vi "InflationApparatus.vi"() -> ()   [LabVIEW 2020]
uses:
  Controls/Outputs.ctl
  <vilib>/userDefined/High Color/IMAQdx.ctl
  Controls/Serpoint.ctl
  Controls/BR2.ctl
  Controls/ButtonEnum.ctl
  Controls/TFspec.ctl
  Controls/Calibration.ctl
  <vilib>/Analysis/6fits.llb/Curve Fitting Criteria.ctl
  <vilib>/DAQmx/read.llb/DAQmx Read (Analog 1D DBL 1Chan NSamp).vi
  <extravilib>/ChannelInstances/Tag-bool/Read With Abort.vi
  <extravilib>/ChannelInstances/Tag-bool/Write With Abort.vi
  <extravilib>/ChannelInstances/Tag-bool/Instantiate.vi
  <extravilib>/ChannelInstances/Tag-bool/EndpointRead.vi
  <extravilib>/ChannelInstances/Tag-bool/Endpoint.vi
  <vilib>/DAQmx/create/channels.llb/DAQmx Create Channel (AI-Voltage-Basic).vi
  <vilib>/DAQmx/configure/timing.llb/DAQmx Timing (Sample Clock).vi
  <vilib>/DAQmx/miscellaneous.llb/DAQmx Fill In Error Info.vi
  <vilib>/Analysis/NI_AALPro.lvlib
  <extravilib>/ChannelInstances/Tag-bool.lvlib
panel:
  in  "Program Stop":bool
  in  "Tab Control":T1(tab)
  in  "Inputs":T4={"File Name"="test.txt", "Force (Hz)"=30.0, "Camera (Hz)"=30.0, "Systole (V)"=0.5, "Diastole (V)"=0.2, "T (sec)"=10.0, "Delay (sec)"=2.0, "Setpoint Function"=enum."Ramp", "Max Diam (mm)"=70.0, "DAQmx Servo Task"="MyPulseOutputTask", "Force Sensor Channel"="Dev2/ai7", "DAQmx LED Task"="MyDigitalOutTask", "Camera Selector"="cam5", "FS Task Out"="", "Servo Task Out"="", "LED Task Out"="", "Camera Session Out"="", "Color Pane"=0} {"Color Pane" items=["Blue", "Red", "Green", "Saturation", "Value", "Intensity", "Luminance", "Hue", ""]}
  in  "ANALYZE":bool
  in  "WRITE TO FILE":bool
  out "Start Time":timestamp
  out "Camera Framerate":dbl(knob) scale=0.0..50.0
  in  "CLEAR \nCHARTS":bool
  in  "Main Start":bool
  out "Diameter (mm)":dbl(graph)
  out "Force Output vs. Setpoint (in Volts)":cluster{"Force Setpoint":dbl, "Force Value":dbl}(graph)
  in  "Main Stop":bool
  out "Camera Buffer":u32
  out "R-Squared":dbl
  out "Outputs":T5
  out "unPWM Signal":dbl[](array[numeric])
  in  "FC Stop":bool
  in  "FC Calculate":bool
  in  "FC Start":bool
  out "Force Sensor Output":dbl(graph)
  in  "FC Log":bool
  out "Calibration Equations":string[][](table)
  out "Calibration Values":string[][](table)
  in  "DAQ Channel":tag="Dev2/ai7"
  in  "Camera Collect":bool
  out "Image":T6(plugin-control)
  in  "Camera Selector":T3
  in  "Settings \n(Clamp (Rake))":T7={"Contrast"=16, "Filter width"=10, "Steepness"=63, "Subsampling Ratio"=30, "Show Search Area"=TRUE, "Show Search Lines"=TRUE, "Show Edges Found"=TRUE, "Show Result"=TRUE}
  out "Framerate":dbl(knob)=4.995836802664447 scale=0.0..100.0
  out "Buffer Number Out":u32=363
  out "Diam (mm)":dbl
  in  "Color Plane":i32(ring)=2 items=["Red", "Green", "Blue", "Hue", "Saturation", "Luminance", "Value", "Intensity"]
  # "Test Variables:"
  # "Sampling Frequencies:"
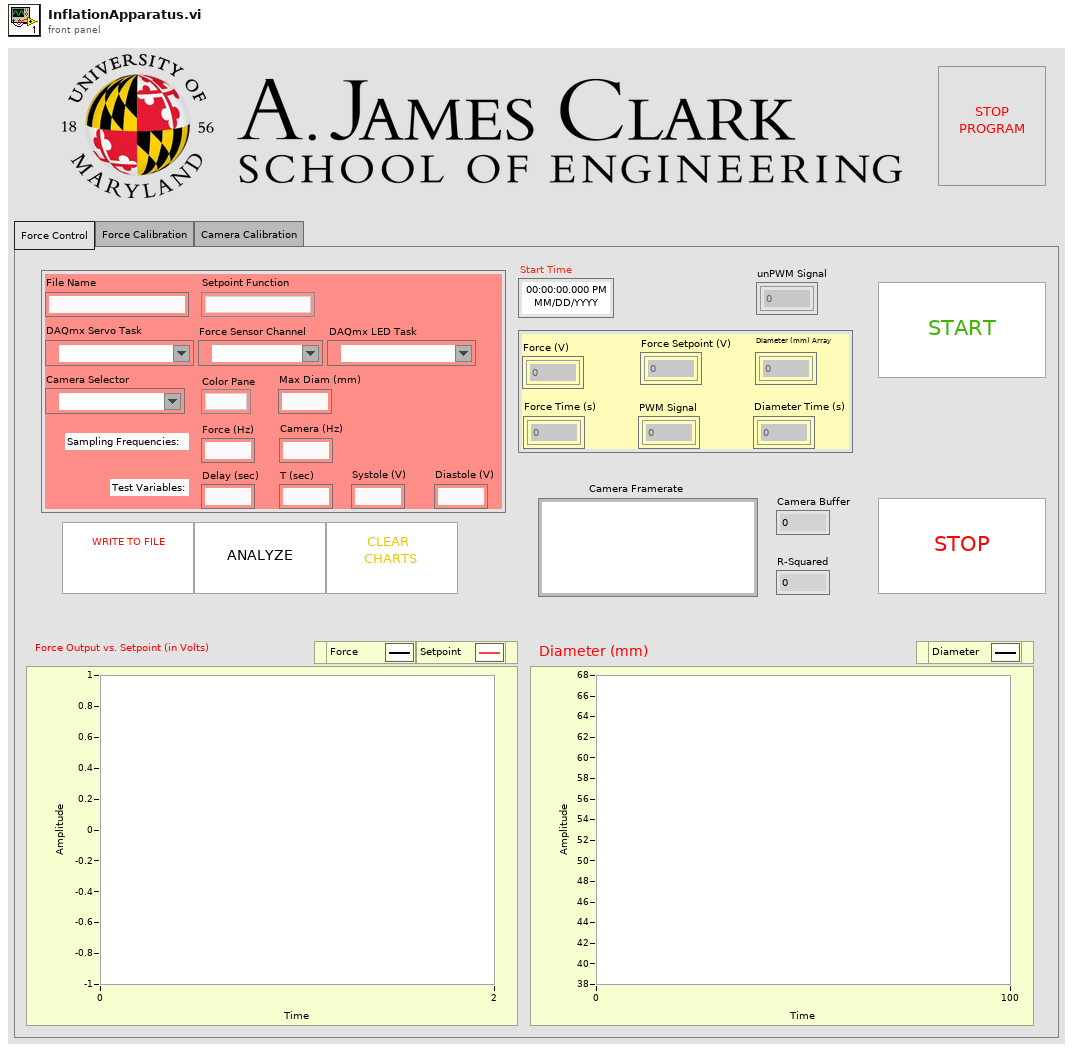
[diagram p1: front panel]
types:
  T1 = enum32{"Force Control", "Force Calibration", "Camera Calibration"}
  T2 = typedef "Serpoint.ctl" = enum16{"Incremental PWM Step", "PWM Step", "Ramp", "Sinusoidal", "Blood-Pressure"}
  T3 = typedef "IMAQdx.ctl" = refnum<k21>
  T4 = cluster{"File Name":string, "Force (Hz)":dbl, "Camera (Hz)":dbl, "Systole (V)":dbl, "Diastole (V)":dbl, "T (sec)":dbl, "Delay (sec)":dbl, "Setpoint Function":T2, "Max Diam (mm)":dbl, "DAQmx Servo Task":refnum<k21>, "Force Sensor Channel":tag, "DAQmx LED Task":refnum<k21>, "Camera Selector":T3, "FS Task Out":refnum<k21>, "Servo Task Out":refnum<k21>, "LED Task Out":refnum<k21>, "Camera Session Out":T3, "Color Pane":i32}
  T5 = typedef "Outputs.ctl" = cluster{"Force Setpoint (V)":dbl[], "PWM Signal":dbl[], "Diameter (mm) Array":dbl[], "Force (V)":dbl[], "Diameter Time (s)":dbl[], "Force Time (s)":dbl[]}
  T6 = typedef "IMAQ Image.ctl" = refnum<image>
  T7 = cluster{"Contrast":i32, "Filter width":i32, "Steepness":i32, "Subsampling Ratio":u32, "Show Search Area":bool, "Show Search Lines":bool, "Show Edges Found":bool, "Show Result":bool}
  T8 = typedef "ButtonEnum.ctl" = enum16{"Initialize", "Analyze", "Clear Charts", "Write to File", "Main Start", "Force Calibration Start", "Force Calibration Calibrate", "Camera Calibration", "Program Stop"}
  T9 = typedef "BR2.ctl" = cluster{"Analyze":refnum<vi>, "Write to File":refnum<vi>, "Clear Charts":refnum<vi>}
  T10 = enum8{"Enabled", "Disabled", "Disabled and Grayed Out"}
  T11 = typedef "TFspec.ctl" = cluster{"b0":dbl, "b1":dbl, "b2":dbl, "a0":dbl, "a1":dbl, "a2":dbl}
  T12 = cluster{"Force Setpoint":dbl, "Force Value":dbl}[]
  T13 = typedef "Inputs.ctl" = cluster{"File Name":string, "Force (Hz)":dbl, "Camera (Hz)":dbl, "Systole (V)":dbl, "Diastole (V)":dbl, "T (sec)":dbl, "Delay (sec)":dbl, "Setpoint Function":T2, "Max Diam (mm)":dbl, "DAQmx Servo Task":refnum<k21>, "Force Sensor Channel":tag, "DAQmx LED Task":refnum<k21>, "Camera Selector":T3, "FS Task Out":refnum<k21>, "Servo Task Out":refnum<k21>, "LED Task Out":refnum<k21>, "Camera Session Out":T3, "Color Pane":i32}
  T14 = typedef "controlspec.ctl" = cluster{"Transfer Function":cluster{"Numerator":dbl[], "Denominator":dbl[]}, "Limit Cluster":cluster{"Upper Limit":dbl, "Lower Limit":dbl}}
  T15 = typedef "ForceCluster.ctl" = cluster{"Force Setpoint":dbl, "PWM Signal":dbl, "Force Value":dbl, "UnPWM Signal":dbl}
  T16 = typedef "Tag-bool.lvlib/))Channel.ctl" = refnum<queue>
  T17 = cluster{"Camera Framerate":dbl, "Camera Buffer":u32, "Diameter (mm)":dbl}
  T18 = typedef "Calibration.ctl" = cluster{"R^2":dbl[], "b":dbl[], "m":dbl[], "CalTable":string[][]}
  T19 = typedef "NI_AALPro.lvlib/Curve Fitting Criteria.ctl" = u16
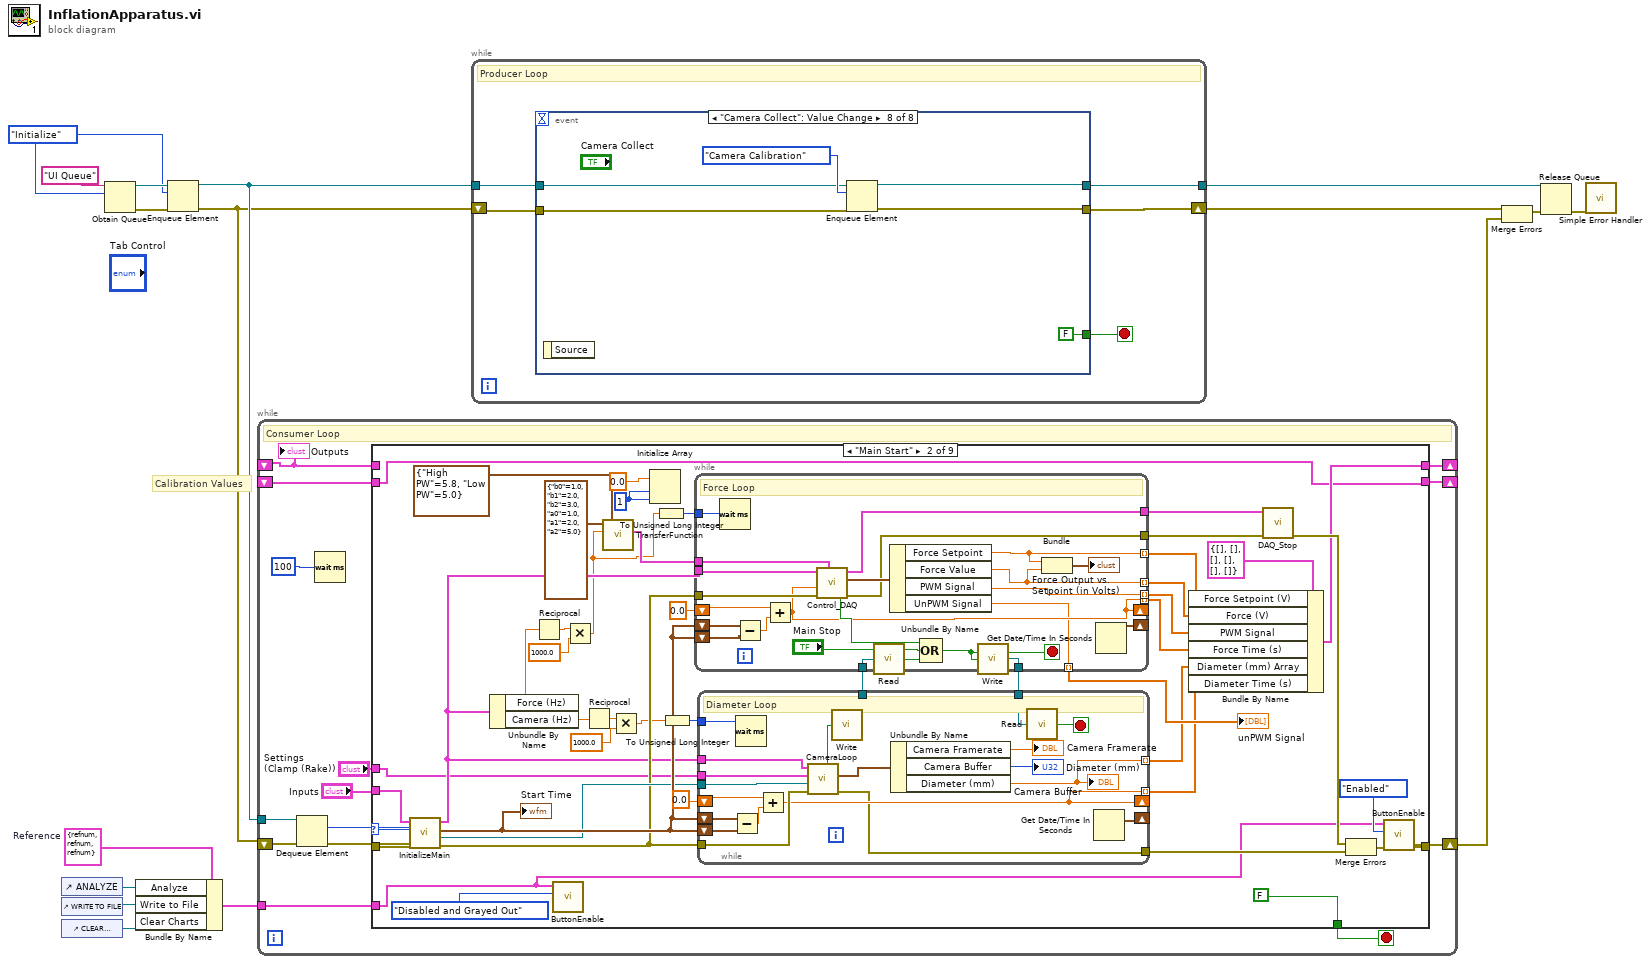
[diagram p0: block diagram]
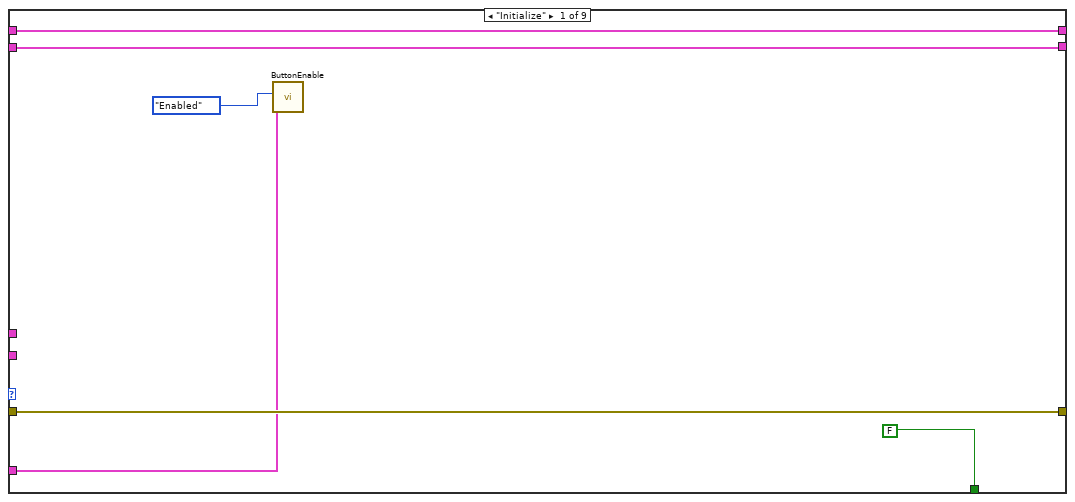
[diagram p2: hidden frame]
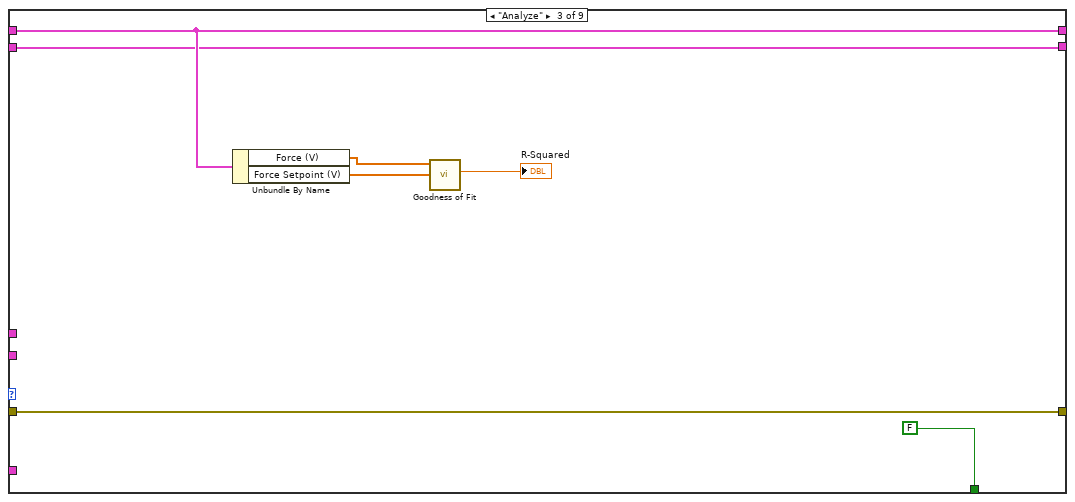
[diagram p3: hidden frame]
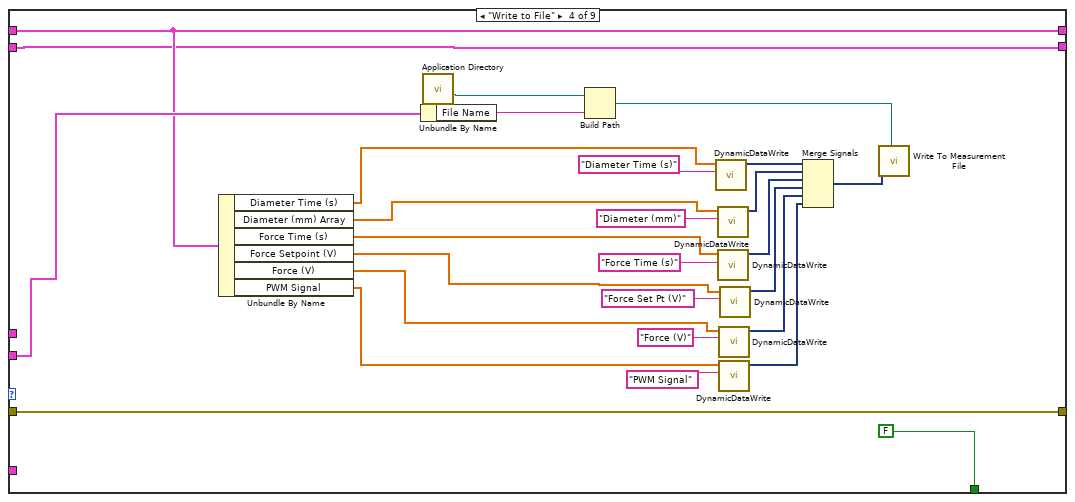
[diagram p4: hidden frame]
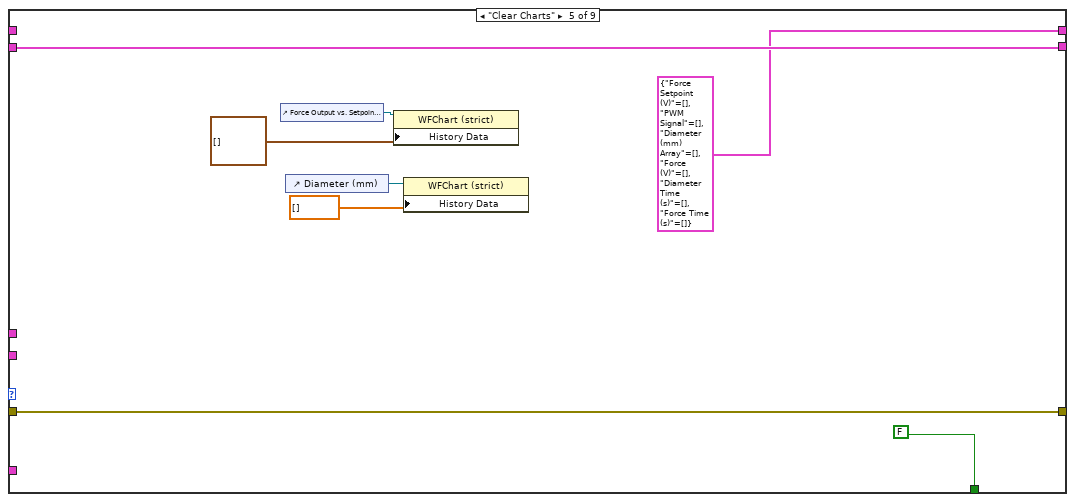
[diagram p5: hidden frame]
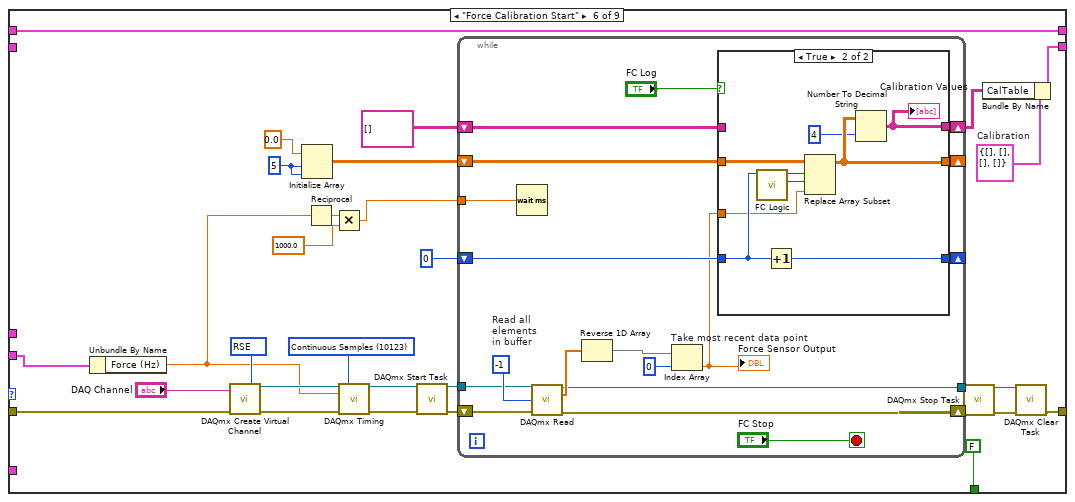
[diagram p6: hidden frame]
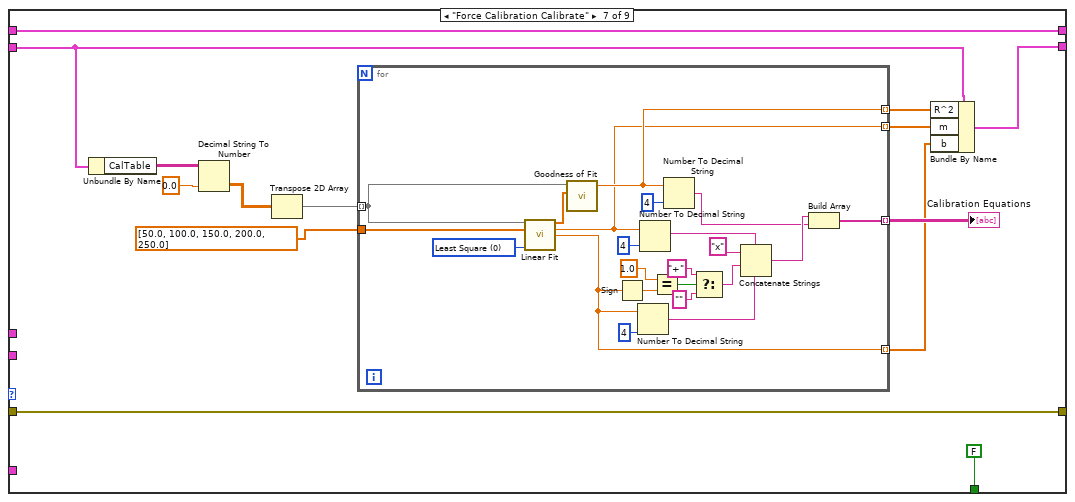
[diagram p8: hidden frame]
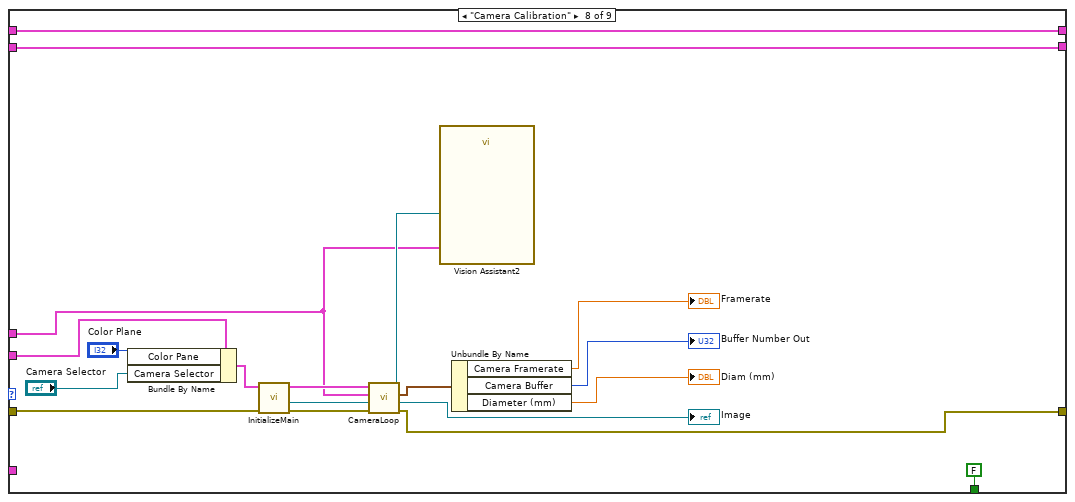
[diagram p9: hidden frame]
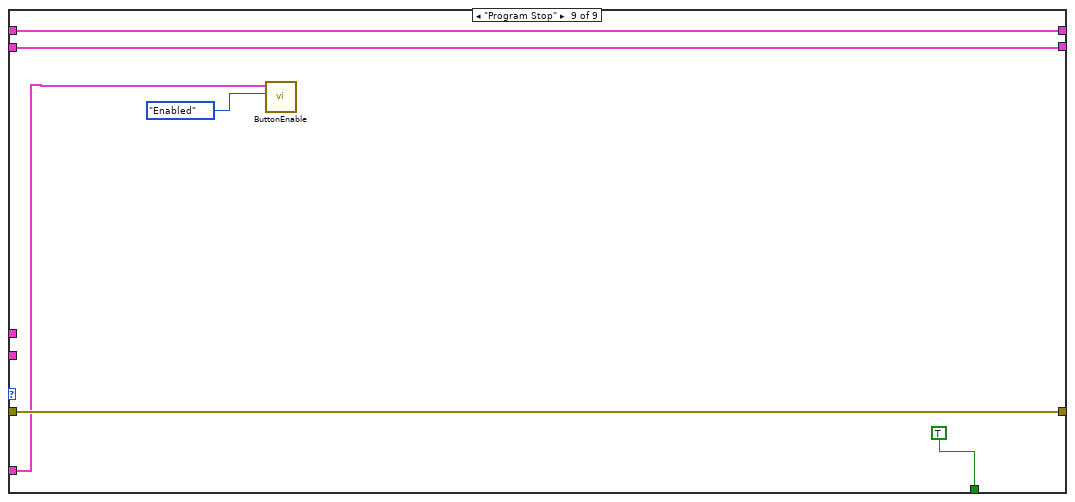
[diagram p10: hidden frame]
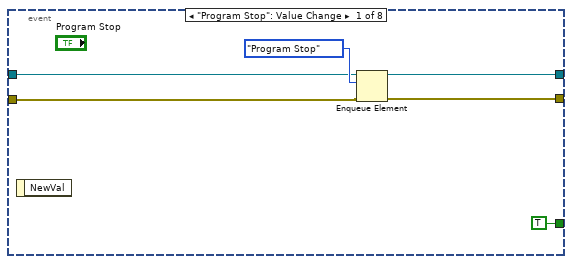
[diagram p11: hidden frame]
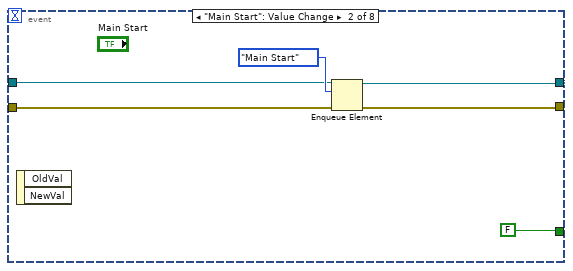
[diagram p12: hidden frame]
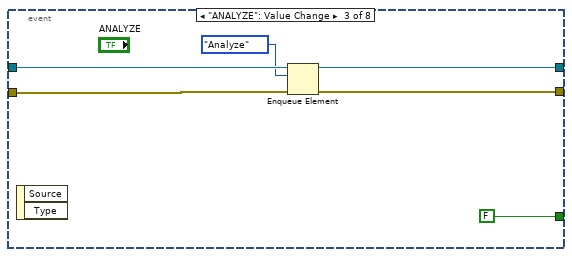
[diagram p13: hidden frame]
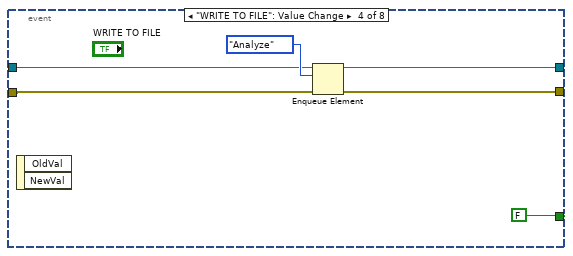
[diagram p14: hidden frame]
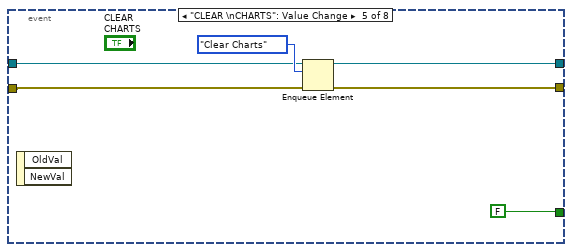
[diagram p15: hidden frame]
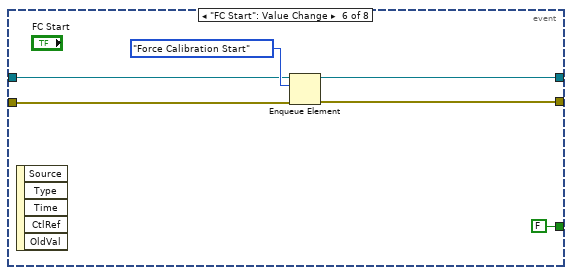
[diagram p16: hidden frame]
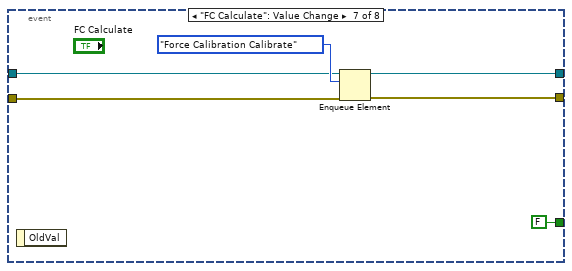
[diagram p17: hidden frame]
diagram:
  w1 = ButtonEnum."Initialize" ("element")
  w13 = T9 {"Analyze"=refnum, "Write to File"=refnum, "Clear Charts"=refnum}  # Reference
  # "Calibration Values"
  n1 = control-ref of="ANALYZE"() -> (w15:refnum<vi>)
  n2 = control-ref of="WRITE TO FILE"() -> (w16:refnum<vi>)
  n3 = control-ref of="CLEAR  CHARTS"() -> (w14:refnum<vi>)
  n4 = Obtain Queue(name (unnamed)="UI Queue", element data type=w1) -> (queue out=w5:refnum<queue>, error out=w4:errorcluster)  [unwired: 3 in, 1 out]
  n5 = Bundle By Name(cluster=w13, "Analyze"=w15, "Write to File"=w16, "Clear Charts"=w14) -> (w11:T9)
  n6 = Enqueue Element(queue=w5, element=w1, error in (no error)=w4) -> (queue out=w3:refnum<queue>, error out=w2:errorcluster)  [unwired: 1 in, 1 out]
  n7 = while {
    tunnel: w3 -> [w29]
    shift-right: [w26] -> w10
    shift-left: w2 -> [w30]
    tunnel: w11 -> [w25]
    shift-right: [w22] -> _
    shift-left: _ -> [w19]
    shift-right: [w21] -> _
    shift-left: _ -> [w20]
    stop <- w23 stop-if-true
    # "Consumer Loop"
    n8 = Dequeue Element(queue=w29, error in (no error)=w30) -> (element=w28:T8, error out=w27:errorcluster)  [unwired: 1 in, 2 out]
    n9 = Wait (ms)(milliseconds to wait=u32 100) -> ()  [unwired: 1 out]
    n10 = case shown="\"Main Start\"" w28 {
      tunnel: w27 -> [w36 w82 w133 w149 w168 w189 w229 w279 w289]
      tunnel: [w36 w37 w133 w149 w168 w182 w229 w275 w289] -> w26
      tunnel: w25 -> [w33 w39 _ _ _ _ _ _ w288]
      tunnel: [FALSE FALSE FALSE FALSE FALSE FALSE FALSE FALSE TRUE] -> w23
      tunnel: "Inputs" -> [_ w78 _ w145 _ w192 _ w271 _]
      tunnel: [w32 w48 w128 w135 T5 {"Force Setpoint (V)"=[], "PWM Signal"=[], "Diameter (mm) Array"=[], "Force (V)"=[], "Diameter Time (s)"=[], "Force Time (s)"=[]} ("Outputs") w197 w242 w270 w285] -> w22
      tunnel: w19 -> [w32 _ w128 w135 _ w197 w242 w270 w285]
      tunnel: [w31 w46 w127 w134 w163 w174 w230 w269 w284] -> w21
      tunnel: w20 -> [w31 w46 w127 w134 w163 _ w234 w269 w284]
      tunnel: "Settings \n(Clamp (Rake))" -> [_ w45 _ _ _ _ _ w265 _]
      frame "Initialize" {
        n11 = call "ButtonEnable.vi"("Disabled"=T10."Enabled", "Reference"=w33) -> ()  [unwired: 9 in, 1 out]
      }
      frame "Main Start" {
        w41 = 1 ("dimension size")
        n12 = call "InitializeMain.vi"("error in"=w82, "Inputs In"=w78) -> ("error out"=w79:errorcluster, "New Image"=w80:T6, "Inputs Out"=w47:T13, "Start Time"=w81:timestamp)  [unwired: 6 in]
        "Start Time" <- w81
        n13 = Unbundle By Name(w47) -> ("Force (Hz)"=w59:dbl, "Camera (Hz)"=w65:dbl)
        n14 = Reciprocal(x=w59) -> (1/x=w61:dbl)
        n15 = call "ButtonEnable.vi"("Disabled"=T10."Disabled and Grayed Out", "Reference"=w39) -> ()  [unwired: 9 in, 1 out]
        n16 = Multiply(x=w61, y=1000.0) -> (x*y=w44:dbl)
        n17 = Reciprocal(x=w65) -> (1/x=w64:dbl)
        n18 = call "TransferFunction.vi"("Limit Cluster"=cluster{"High PW":dbl, "Low PW":dbl} {"High PW"=5.8, "Low PW"=5.0}, "Sampling Time (s)"=w44, "Cluster"=T11 {"b0"=1.0, "b1"=2.0, "b2"=3.0, "a0"=1.0, "a1"=2.0, "a2"=5.0}) -> ("Transfer Function"=w56:T14)  [unwired: 6 in, 2 out]
        n19 = Multiply(x=w64, y=1000.0) -> (x*y=w62:dbl)
        n20 = Initialize Array(0.0 ("element"), w41, w41) -> ()  [unwired: 1 out]
        n21 = To Unsigned Long Integer(number=w44) -> (unsigned 32bit integer=w43:u32)
        n22 = To Unsigned Long Integer(number=w62) -> (unsigned 32bit integer=w73:u32)
        n23 = while {
          shift-right: [w126] -> _
          shift-left: w81 -> [w123]
          shift-left: w81 -> [w124]
          shift-right: [w113] -> _
          shift-left: 0.0 -> [w122]
          tunnel: w47 -> [w121]
          tunnel: w79 -> [w120]
          tunnel: w72 -> [w119]
          tunnel: [w114] -> w71
          tunnel: [w113] -> w51 mode=indexing
          tunnel: [w111] -> w52 mode=indexing
          tunnel: [w104] -> w53 mode=indexing
          tunnel: [w110] -> w70
          tunnel: [w109] -> w69
          tunnel: [w103] -> w54 mode=indexing
          tunnel: [w108] -> w58 mode=indexing
          tunnel: w56 -> [w107]
          tunnel: w43 -> [w106]
          stop <- w115 stop-if-true
          # "Force Loop"
          n24 = Wait (ms)(milliseconds to wait=w106) -> ()  [unwired: 1 out]
          n25 = Subtract(x=w123, y=w124) -> (x-y=w125:dbl)
          n26 = Add(x=w122, y=w125) -> (x+y=w113:dbl)
          n27 = call "Control_DAQ.vi"("Transfer Function"=w107, "error in"=w120, "Time"=w113, "Inputs"=w121) -> ("error out"=w110:errorcluster, "Force cluster"=w112:T15, "Inputs Out"=w109:T13, "Time Exceeded?"=w116:bool)  [unwired: 4 in]
          n28 = call <extravilib>:"Read.vi"("channel"=w119) -> ("element"=w118:bool)  [unwired: 1 in, 1 out]
          n29 = Unbundle By Name(w112) -> ("Force Setpoint"=w103:dbl, "Force Value"=w104:dbl, "PWM Signal"=w111:dbl, "UnPWM Signal"=w108:dbl)
          n30 = Compound Arithmetic op=OR(w116, "Main Stop", w118) -> (w115:bool)
          n31 = call <extravilib>:"Write.vi"("element"=w115) -> ("channel"=w114:T16)  [unwired: 1 out]
          n32 = Bundle("Force Setpoint"=w103, "Force Value"=w104) -> (→"Force Output vs. Setpoint (in Volts)":cluster{"Force Setpoint":dbl, "Force Value":dbl})  [unwired: 1 in]
          n33 = Get Date/Time In Seconds() -> (seconds since 1Jan1904=w126:timestamp)
        }
        "unPWM Signal" <- w58
        n34 = while {
          shift-right: [w102] -> _
          shift-left: w81 -> [w101]
          shift-left: w81 -> [w100]
          shift-right: [w85] -> _
          shift-left: 0.0 -> [w98]
          tunnel: w79 -> [w97]
          tunnel: w80 -> [w96]
          tunnel: w47 -> [w95]
          tunnel: w73 -> [w94]
          tunnel: [w90] -> w50 mode=indexing
          tunnel: [w88] -> w72
          tunnel: w71 -> [w87]
          tunnel: [w85] -> w49 mode=indexing
          tunnel: [w84] -> w68
          tunnel: w45 -> [w83]
          stop <- w86 stop-if-true
          # "Diameter Loop"
          n35 = Subtract(x=w101, y=w100) -> (x-y=w99:dbl)
          n36 = Wait (ms)(milliseconds to wait=w94) -> ()  [unwired: 1 out]
          n37 = Add(x=w98, y=w99) -> (x+y=w85:dbl)
          n38 = call "CameraLoop.vi"("error in"=w97, "Image In"=w96, "Settings (Clamp (Rake))"=w83, "Inputs"=w95) -> ("error out"=w84:errorcluster, "Diameter Cluster"=w93:T17, "Diameter Exceeded?"=w89:bool)  [unwired: 3 in, 2 out]
          n39 = call <extravilib>:"Write.vi"("element"=w89) -> ("channel"=w88:T16)  [unwired: 1 out]
          n40 = Unbundle By Name(w93) -> ("Camera Framerate"=→"Camera Framerate":dbl, "Camera Buffer"=→"Camera Buffer":u32, "Diameter (mm)"=w90:dbl)
          "Diameter (mm)" <- w90
          n41 = call <extravilib>:"Read.vi"("channel"=w87) -> ("element"=w86:bool)  [unwired: 1 in, 1 out]
          n42 = Get Date/Time In Seconds() -> (seconds since 1Jan1904=w102:timestamp)
        }
        n43 = Bundle By Name(cluster=T5 {"Force Setpoint (V)"=[], "PWM Signal"=[], "Diameter (mm) Array"=[], "Force (V)"=[], "Diameter Time (s)"=[], "Force Time (s)"=[]} ("Outputs"), "Force Setpoint (V)"=w54, "Force (V)"=w53, "PWM Signal"=w52, "Force Time (s)"=w51, "Diameter (mm) Array"=w50, "Diameter Time (s)"=w49) -> (w48:T5)
        n44 = call "DAQ_Stop.vi"("error in (no error)"=w70, "Inputs"=w69) -> ("error out"=w67:errorcluster)  [unwired: 9 in]
        n45 = Merge Errors(w67, w68) -> (w38:errorcluster)
        n46 = call "ButtonEnable.vi"("error in"=w38, "Disabled"=T10."Enabled", "Reference"=w39) -> ("error out"=w37:errorcluster)  [unwired: 8 in]
      }
      frame "Analyze" {
        n47 = Unbundle By Name(w128) -> ("Force (V)"=w130:dbl[], "Force Setpoint (V)"=w129:dbl[])
        n48 = call <vilib>:"Goodness of Fit.vi"("Best Fit"=w129, "Y"=w130) -> ("R-square"=→"R-Squared":dbl)  [unwired: 6 in, 3 out]
      }
      frame "Write to File" {
        n49 = Unbundle By Name(w135) -> ("Diameter Time (s)"=w141:dbl[], "Diameter (mm) Array"=w140:dbl[], "Force Time (s)"=w139:dbl[], "Force Setpoint (V)"=w138:dbl[], "Force (V)"=w136:dbl[], "PWM Signal"=w137:dbl[])
        n50 = Unbundle By Name(w145) -> ("File Name"=w143:string)
        n51 = call <vilib>:"Application Directory.vi"() -> ("Application Directory"=w144:path)
        n52 = Build Path(base path=w144, name or relative path=w143) -> (appended path=w142:path)
        n53 = call "DynamicDataWrite"("String"="Diameter Time (s)", "Array"=w141) -> ("Signals Out"=w159:dynamicdata)  [unwired: 9 in]
        n54 = call "DynamicDataWrite"("String"="Diameter (mm)", "Array"=w140) -> ("Signals Out"=w158:dynamicdata)  [unwired: 9 in]
        n55 = call "DynamicDataWrite"("String"="Force Time (s)", "Array"=w139) -> ("Signals Out"=w157:dynamicdata)  [unwired: 9 in]
        n56 = call "DynamicDataWrite"("String"="Force (V)", "Array"=w136) -> ("Signals Out"=w155:dynamicdata)  [unwired: 9 in]
        n57 = call "DynamicDataWrite"("String"="PWM Signal", "Array"=w137) -> ("Signals Out"=w146:dynamicdata)  [unwired: 9 in]
        n58 = call "DynamicDataWrite"("String"="Force Set Pt (V)", "Array"=w138) -> ("Signals Out"=w156:dynamicdata)  [unwired: 9 in]
        n59 = Merge Signals(w159, w158, w157, w156, w155, w146) -> (w160:dynamicdata)
        n60 = call "Write To Measurement File"("Signals"=w160, "Filename"=w142) -> ()  [unwired: 15 in, 3 out]
      }
      frame "Clear Charts" {
        n61 = control-ref of="Force Output vs. Setpoint (in Volts)"() -> (w165:refnum<vi>)
        n62 = control-ref of="Diameter (mm)"() -> (w167:refnum<vi>)
        n63 = property class="WFChart (strict)"(reference=w165, "History Data"=T12 []) -> ()  [unwired: 1 in, 2 out]
        n64 = property class="WFChart (strict)"(reference=w167, "History Data"=dbl[] []) -> ()  [unwired: 1 in, 2 out]
      }
      frame "Force Calibration Start" {
        w175 = T18 {"R^2"=[], "b"=[], "m"=[], "CalTable"=[]}  # Calibration
        w180 = 5 ("dimension size")
        w194 = 10083 items=["Default"=-1, "RSE"=10083, "NRSE"=10078, "Differential"=10106, "Pseudodifferential"=12529] ("input terminal configuration")
        w193 = 10123 items=["Finite Samples"=10178, "Continuous Samples"=10123, "Hardware Timed Single Point"=12522] ("sample mode")
        n65 = Unbundle By Name(w192) -> ("Force (Hz)"=w171:dbl)
        n66 = call-poly <vilib>:"DAQmx Create Virtual Channel.vi"("input terminal configuration"=w194, "physical channels"="DAQ Channel", "error in"=w189) -> ("task out"=w195:refnum<k21>, "error out"=w196:errorcluster)  [unwired: 11 in]
        n67 = Initialize Array(0.0 ("element"), w180, w180) -> (w179:dbl[][])
        n68 = Reciprocal(x=w171) -> (1/x=w172:dbl)
        n69 = Multiply(x=w172, y=1000.0) -> (x*y=w169:dbl)
        n70 = call-poly <vilib>:"DAQmx Timing.vi"("task/channels in"=w195, "sample mode"=w193, "rate"=w171, "error in"=w196) -> ("task out"=w191:refnum<k21>, "error out"=w190:errorcluster)  [unwired: 10 in]
        n71 = call <vilib>:"DAQmx Start Task.vi"("task/channels in"=w191, "error in"=w190) -> ("task out"=w188:refnum<k21>, "error out"=w187:errorcluster)  [unwired: 12 in]
        n72 = while {
          tunnel: w188 -> [w211]
          tunnel: [w209] -> w184
          shift-right: [w208] -> w183
          shift-left: w187 -> [w210]
          shift-right: [w205] -> _
          shift-left: w179 -> [w206]
          shift-right: [w203] -> _
          shift-left: 0 -> [w204]
          shift-right: [w201] -> w176
          shift-left: string[][] [] -> [w200]
          tunnel: w169 -> [w199]
          stop <- "FC Stop" stop-if-true
          w215 = -1  # Read all elements in buffer
          n73 = Wait (ms)(milliseconds to wait=w199) -> ()  [unwired: 1 out]
          n74 = call-poly <vilib>:"DAQmx Read.vi"("task/channels in"=w211, "number of samples per channel"=w215, "error in"=w210) -> ("task out"=w209:refnum<k21>, "data"=w214:dbl[], "error out"=w208:errorcluster)  [unwired: 10 in]
          n75 = Reverse 1D Array(array=w214) -> (reversed array=w213:dbl[])
          n76 = Index Array "Take most recent data point"(array=w213, index=0) -> (element=w202:dbl)
          "Force Sensor Output" <- w202
          n77 = case shown="True" "FC Log" {
            tunnel: w206 -> [w219 w228]
            tunnel: [w219 w222] -> w205
            tunnel: w204 -> [w218 w226]
            tunnel: [w218 w227] -> w203
            tunnel: w202 -> [_ w223]
            tunnel: [w217 w220] -> w201
            tunnel: w200 -> [w217 _]
            frame False {
            }
            frame True {
              n78 = call "FC Logic.vi"("Log Iteration"=w226) -> ("Column"=w224:i32, "Row"=w225:i32)  [unwired: 9 in]
              n79 = Increment(x=w226) -> (x+1=w227:i32)
              n80 = Replace Array Subset(array=w228, new element=w223, index (row)=w225, index (col)=w224) -> (w222:dbl[][])
              n81 = Number To Decimal String(number=w222, width (-)=i16 4) -> (decimal integer string=w220:string[][])
              "Calibration Values" <- w220
            }
          }
        }
        n82 = call <vilib>:"DAQmx Stop Task.vi"("task/channels in"=w184, "error in"=w183) -> ("task out"=w185:refnum<k21>, "error out"=w186:errorcluster)  [unwired: 12 in]
        n83 = Bundle By Name(cluster=w175, "CalTable"=w176) -> (w174:T18)
        n84 = call <vilib>:"DAQmx Clear Task.vi"("task in"=w185, "error in"=w186) -> ("error out"=w182:errorcluster)  [unwired: 13 in]
      }
      frame "Force Calibration Calibrate" {
        n85 = Unbundle By Name(w234) -> ("CalTable"=w235:string[][])
        n86 = Decimal String To Number(string=w235, default (0L)=0.0 ("default (0 I32)")) -> (number=w239:dbl[][])  [unwired: 1 in, 1 out]
        n87 = Transpose 2D Array(2D array=w239) -> (transposed array=w238:dbl[][])
        n88 = for {
          tunnel: w238 -> [w262] mode=indexing
          tunnel: dbl[] [50.0, 100.0, 150.0, 200.0, 250.0] -> [w263]
          tunnel: [w246] -> w236 mode=indexing
          tunnel: [w245] -> w233 mode=indexing
          tunnel: [w244] -> w232 mode=indexing
          tunnel: [w243] -> w231 mode=indexing
          w264 = T19 0 items=["Least Square", "Least Absolute Residual", "Bisquare"] ("method")
          n89 = call <vilib>:"Linear Fit.vi"("Y"=w262, "X"=w263, "method"=w264) -> ("Best Linear Fit"=w261:dbl[], "slope"=w244:dbl, "intercept"=w243:dbl)  [unwired: 8 in, 2 out]
          n90 = call <vilib>:"Goodness of Fit.vi"("Best Fit"=w261, "Y"=w262) -> ("R-square"=w245:dbl)  [unwired: 6 in, 3 out]
          n91 = Sign(1:w243) -> (0:w254:dbl)
          n92 = Number To Decimal String(number=w243, width (-)=i16 4) -> (decimal integer string=w255:string)
          n93 = Number To Decimal String(number=w244, width (-)=i16 4) -> (decimal integer string=w256:string)
          n94 = Equal?(x=1.0, y=w254) -> (x = y?=w252:bool)
          n95 = Number To Decimal String(number=w245, width (-)=i16 4) -> (decimal integer string=w247:string)
          n96 = Select(t="+" ("string"), s=w252, f="" ("string")) -> (s? t:f=w249:string)
          n97 = Concatenate Strings(w256, "x" ("string"), w249, w255) -> (w248:string)
          n98 = Build Array(w248, w247) -> (w246:string[])
        }
        "Calibration Equations" <- w236
        n99 = Bundle By Name(cluster=w234, "R^2"=w233, "m"=w232, "b"=w231) -> (w230:T18)
      }
      frame "Camera Calibration" {
        n100 = Bundle By Name(cluster=w271, "Color Pane"="Color Plane", "Camera Selector"="Camera Selector") -> (w267:T4)
        n101 = call "InitializeMain.vi"("error in"=w279, "Inputs In"=w267) -> ("error out"=w280:errorcluster, "New Image"=w282:T6, "Inputs Out"=w281:T13)  [unwired: 6 in, 1 out]
        n102 = call "CameraLoop.vi"("error in"=w280, "Image In"=w282, "Settings (Clamp (Rake))"=w265, "Inputs"=w281) -> ("error out"=w275:errorcluster, "Image Out"=→"Image":T6, "Diameter Cluster"=w283:T17, "Image Dst Out"=w266:T6)  [unwired: 3 in, 1 out]
        n103 = call "Vision Assistant2"("Image In"=w266, "Settings (Clamp (Rake) 1)"=w265) -> ()  [unwired: 22 in, 4 out]
        n104 = Unbundle By Name(w283) -> ("Camera Framerate"=→"Framerate":dbl, "Camera Buffer"=→"Buffer Number Out":u32, "Diameter (mm)"=→"Diam (mm)":dbl)
      }
      frame "Program Stop" {
        n105 = call "ButtonEnable.vi"("Disabled"=T10."Enabled", "Reference"=w288) -> ()  [unwired: 9 in, 1 out]
      }
    }
    "Outputs" <- w19
  }
  n106 = while {
    tunnel: w3 -> [w293]
    tunnel: [w290] -> w7
    shift-right: [w291] -> w9
    shift-left: w2 -> [w292]
    stop <- w294 stop-if-true
    # "Producer Loop"
    n107 = event shown="[7] \"Camera Collect\": Value Change" {
      selector: _ -> [_ _ _ _ _ _ _ _]
      dyn-events: _ -> [_ _ _ _ _ _ _ _]
      timeout: _ -> [_ _ _ _ _ _ _ _]
      tunnel: [TRUE FALSE FALSE FALSE FALSE FALSE FALSE FALSE] -> w294
      tunnel: w293 -> [w299 w304 w311 w316 w322 w329 w335 w340]
      tunnel: w292 -> [w298 w303 w310 w315 w321 w328 w334 w339]
      tunnel: [w297 w301 w309 w314 w320 w327 w333 w338] -> w290
      tunnel: [w296 w302 w308 w313 w319 w326 w332 w337] -> w291
      event "Program Stop": Value Change {
        n108 = event-data() -> ()  [unwired: 1 in, 1 out]
        n109 = Enqueue Element(queue=w299, element=ButtonEnum."Program Stop", error in (no error)=w298) -> (queue out=w297:refnum<queue>, error out=w296:errorcluster)  [unwired: 1 in, 1 out]
      }
      event "Main Start": Value Change {
        n110 = event-data() -> ()  [unwired: 1 in, 2 out]
        n111 = Enqueue Element(queue=w304, element=ButtonEnum."Main Start", error in (no error)=w303) -> (queue out=w301:refnum<queue>, error out=w302:errorcluster)  [unwired: 1 in, 1 out]
      }
      event "ANALYZE": Value Change {
        n112 = event-data() -> ()  [unwired: 1 in, 2 out]
        n113 = Enqueue Element(queue=w311, element=ButtonEnum."Analyze", error in (no error)=w310) -> (queue out=w309:refnum<queue>, error out=w308:errorcluster)  [unwired: 1 in, 1 out]
      }
      event "WRITE TO FILE": Value Change {
        n114 = event-data() -> ()  [unwired: 1 in, 2 out]
        n115 = Enqueue Element(queue=w316, element=ButtonEnum."Analyze", error in (no error)=w315) -> (queue out=w314:refnum<queue>, error out=w313:errorcluster)  [unwired: 1 in, 1 out]
      }
      event "CLEAR \nCHARTS": Value Change {
        n116 = event-data() -> ()  [unwired: 1 in, 2 out]
        n117 = Enqueue Element(queue=w322, element=ButtonEnum."Clear Charts", error in (no error)=w321) -> (queue out=w320:refnum<queue>, error out=w319:errorcluster)  [unwired: 1 in, 1 out]
      }
      event "FC Start": Value Change {
        n118 = event-data() -> ()  [unwired: 1 in, 5 out]
        n119 = Enqueue Element(queue=w329, element=ButtonEnum."Force Calibration Start", error in (no error)=w328) -> (queue out=w327:refnum<queue>, error out=w326:errorcluster)  [unwired: 1 in, 1 out]
      }
      event "FC Calculate": Value Change {
        n120 = event-data() -> ()  [unwired: 1 in, 1 out]
        n121 = Enqueue Element(queue=w335, element=ButtonEnum."Force Calibration Calibrate", error in (no error)=w334) -> (queue out=w333:refnum<queue>, error out=w332:errorcluster)  [unwired: 1 in, 1 out]
      }
      event "Camera Collect": Value Change {
        n122 = event-data() -> ()  [unwired: 1 in, 1 out]
        n123 = Enqueue Element(queue=w340, element=ButtonEnum."Camera Calibration", error in (no error)=w339) -> (queue out=w338:refnum<queue>, error out=w337:errorcluster)  [unwired: 1 in, 1 out]
      }
    }
  }
  n124 = Merge Errors(w9, w10) -> (w8:errorcluster)
  n125 = Release Queue(queue=w7, error in (no error)=w8) -> (error out=w6:errorcluster)  [unwired: 1 in, 2 out]
  n126 = call <vilib>:"Simple Error Handler.vi"("error in (no error)"=w6) -> ()  [unwired: 4 in, 5 out]
